vi "FPGA_PWM_dc_motor.vi"(7 "DC PWM Frequency (Hz)":sgl=20000.0, 8 "Encoder Debug":bool, 9 "Loop Timer DAQ":u32=1 caption="Loop Time(uSec)", 10 "Velocity Interval (uSec)":u32=1000, 11 "Controller PWM output [-100,100]%":sgl(slide) scale=-100.0..100.0) -> (0 "Acceleration (Counts/Interval)":i32, 1 "Velocity (Counts/Interval)":i32, 3 "Position (Counts)":i64)   [LabVIEW 2019]
uses:
  <vilib>/rvi/Emulation/niFpgaSctlEmulationGetInTimedLoop.vi
  <vilib>/rvi/Emulation/niFpgaProcessEmulError.vi
  <vilib>/rvi/Emulation/niFpgaGetClockAttributes.vi
  <vilib>/rvi/Emulation/niFpgaEmulationReportErrorSimple.vi
  <vilib>/rvi/eio/common/nirviEmuTemplateMethod_errors.vi
  <vilib>/rvi/Emulation/niFpgaCriticalErrorInLSC.vi
  <vilib>/eio/EIONode/EIONode.xnode
panel:
  out "ConnectorA/DIO13":bool
  out "ConnectorA/DIO12":bool
  in  "Debug: ConnectorA/DIO15":bool
  in  "Debug: ConnectorA/DIO14":bool
  in  "Position Reset":bool
  out "B":bool
  out "A":bool
  out "B'":bool
  out "A'":bool
  in  "stop":bool
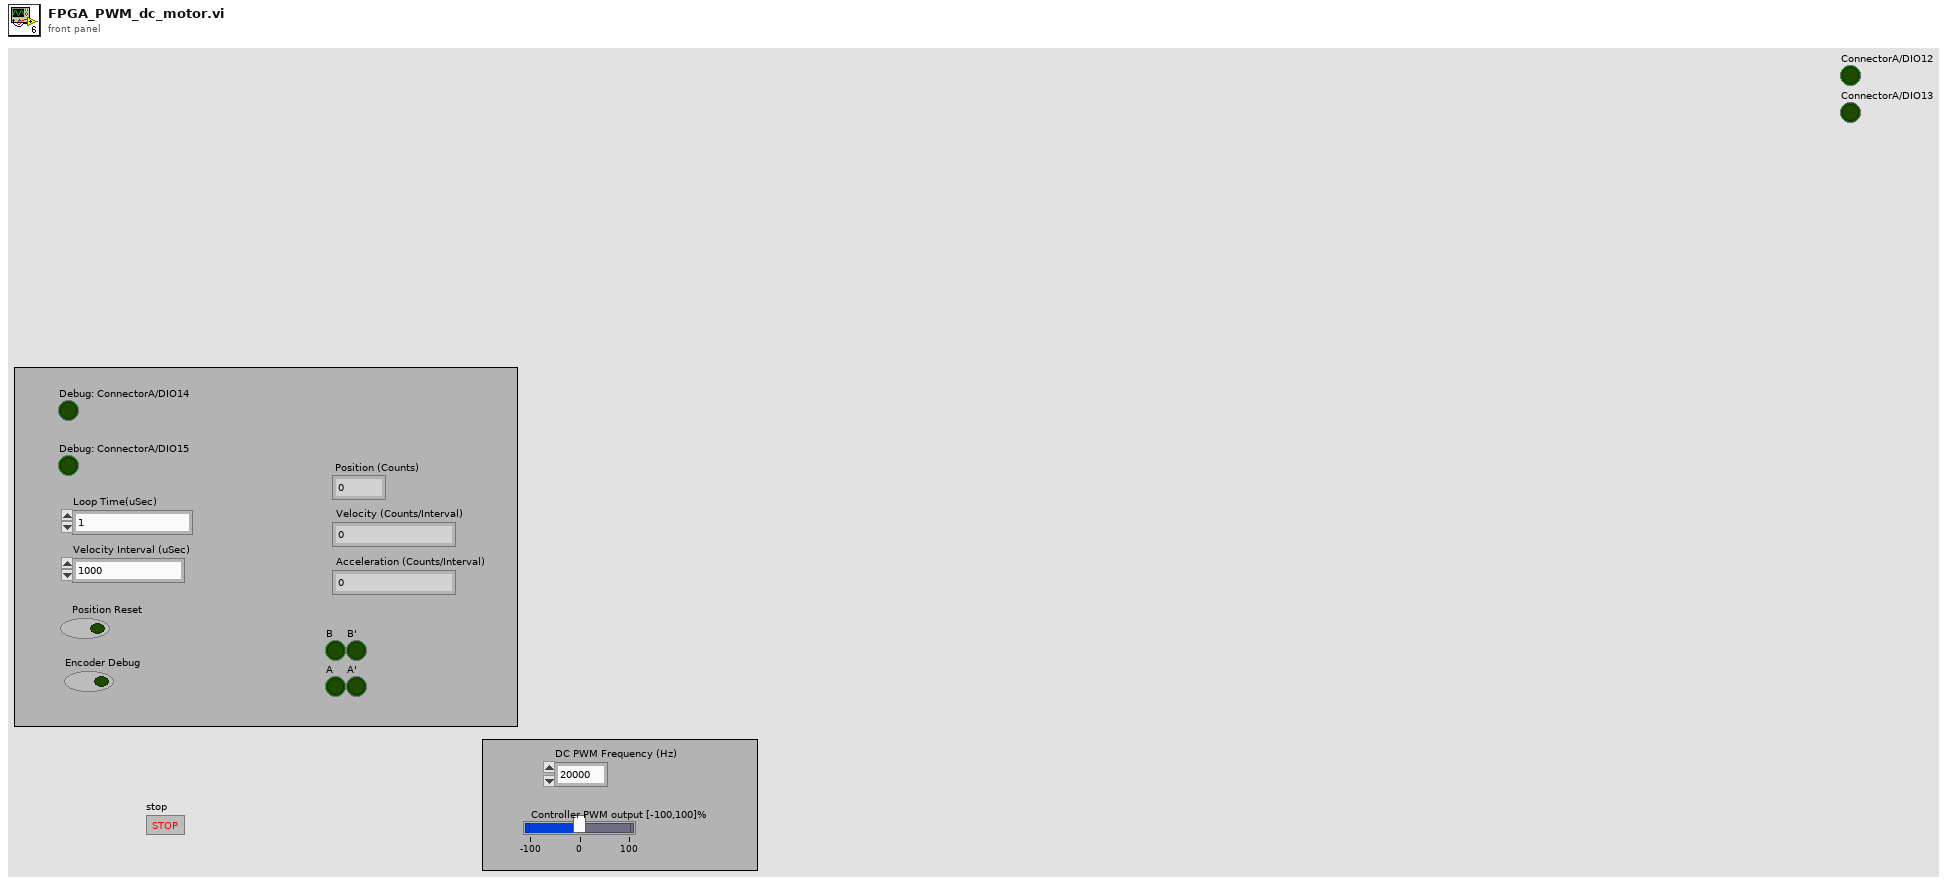
[diagram p1: front panel]
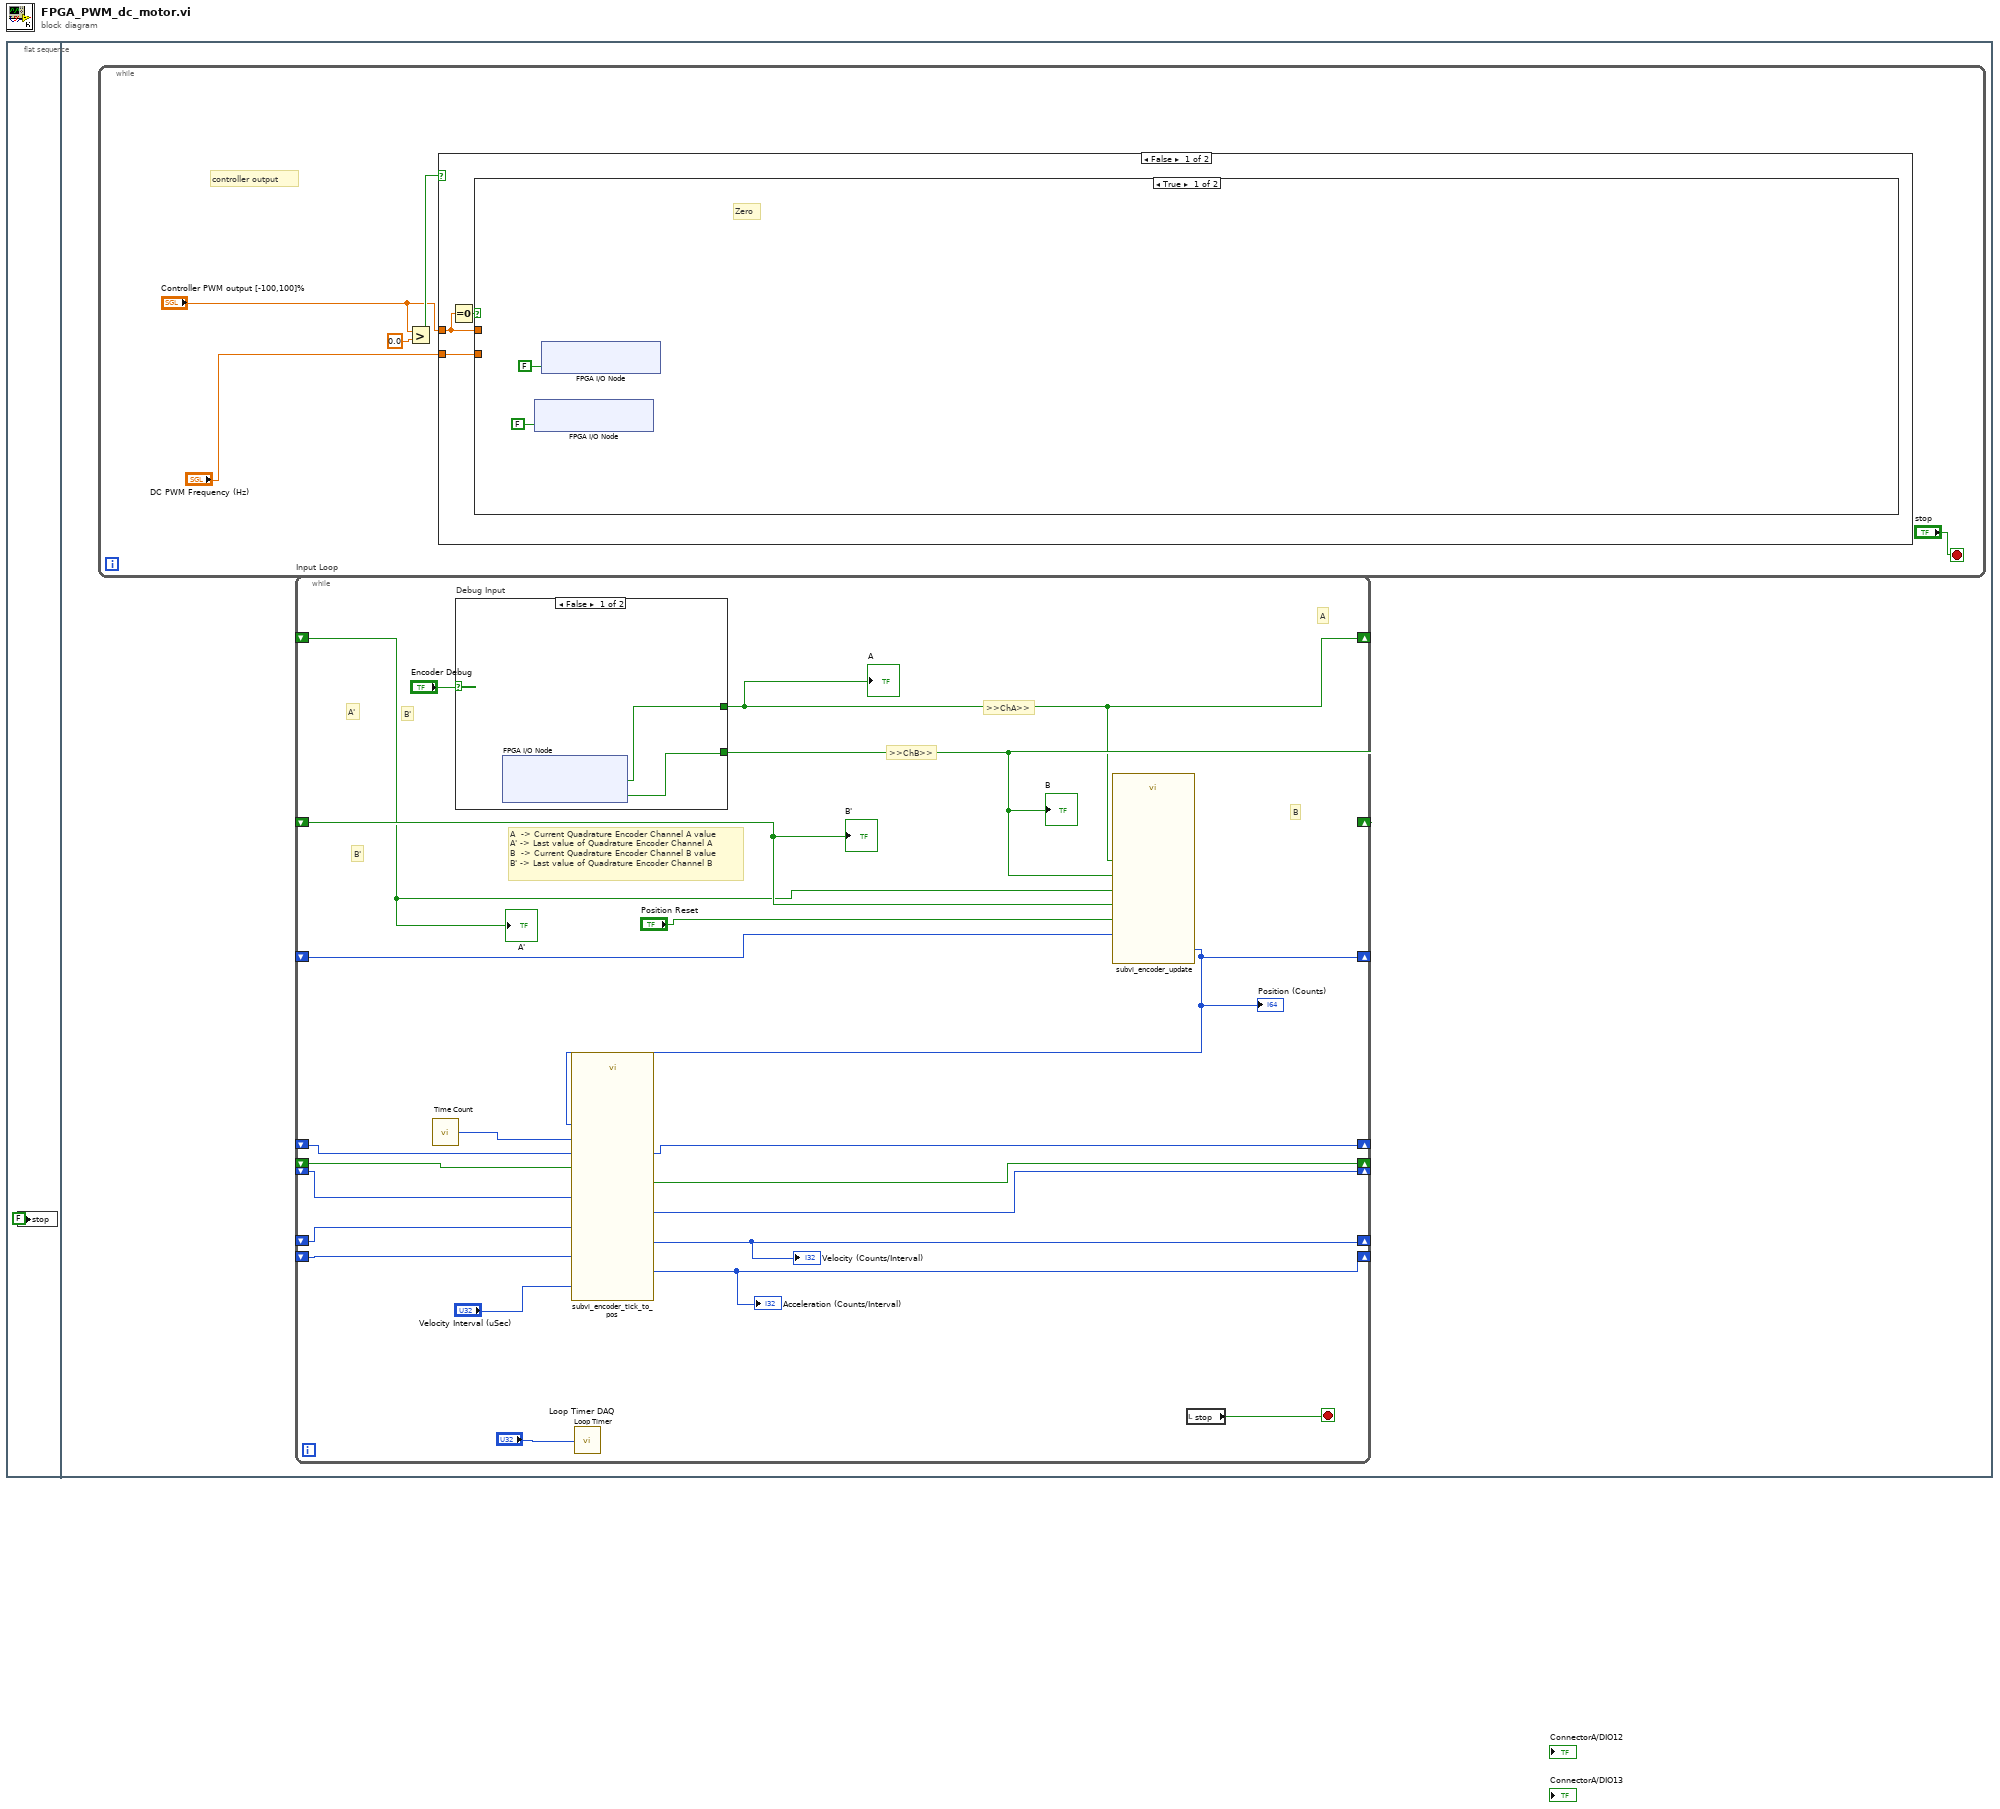
[diagram p0: block diagram]
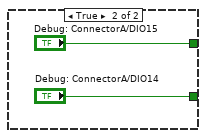
[diagram p2: hidden frame]
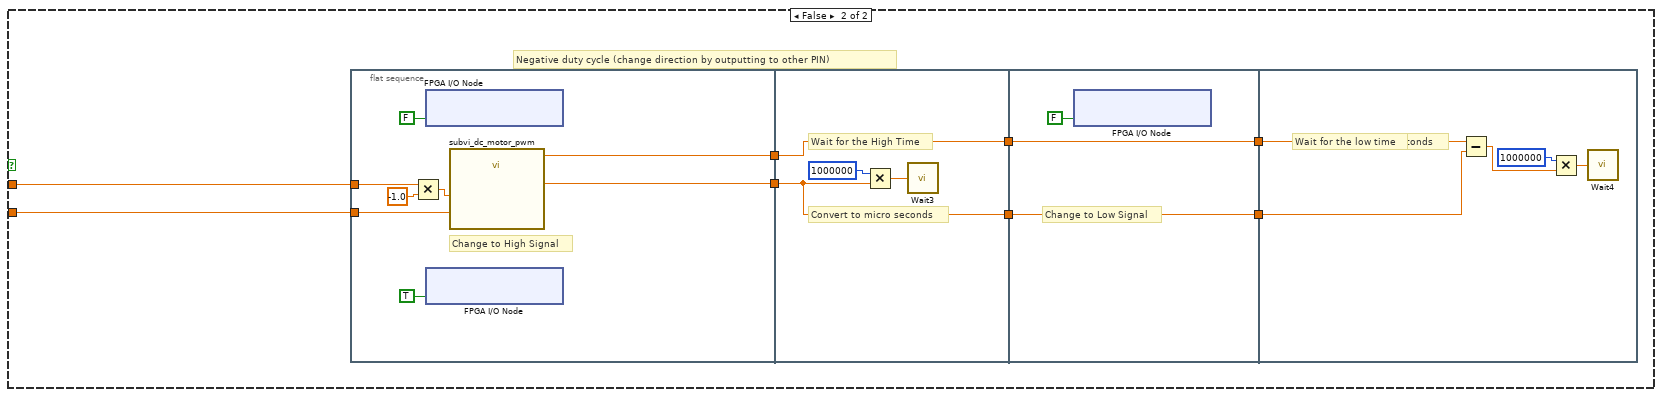
[diagram p3: hidden frame]
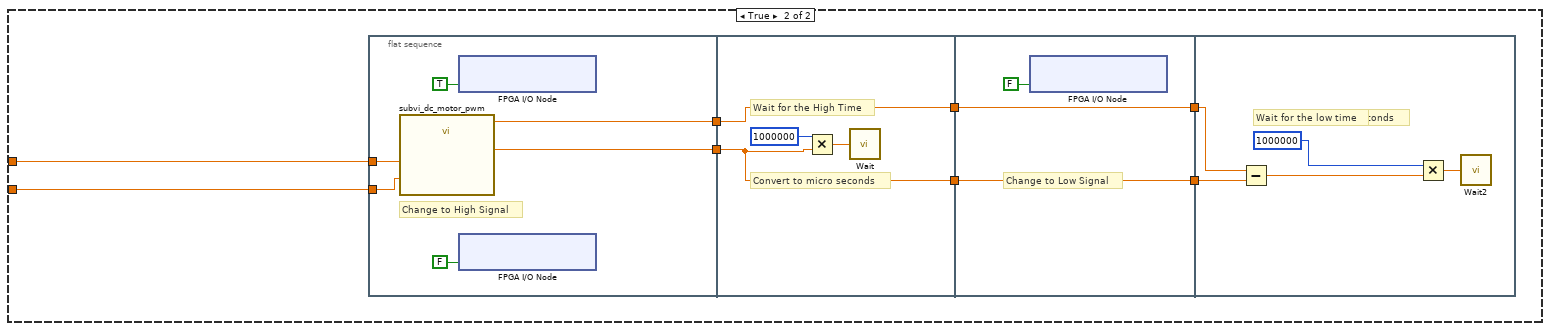
[diagram p4: hidden frame]
diagram:
  n1 = flat-sequence {
    frame #0 {
      n2 = local write "stop"(FALSE ("stop")) -> ()
    }
    frame #1 {
      n3 = while {
        stop <- "stop" stop-if-true
        # "controller output"
        n4 = Greater?(x="Controller PWM output [-100,100]%", y=sgl 0.0) -> (0:w29:bool)
        n5 = case shown="False" w29 {
          tunnel: "DC PWM Frequency (Hz)" -> [w35 w67]
          tunnel: "Controller PWM output [-100,100]%" -> [w34 w66]
          frame False {
            n6 = Equal To 0?(x=w34) -> (x = 0?=w33:bool)
            n7 = case shown="True" w33 {
              tunnel: w34 -> [_ w39]
              tunnel: w35 -> [_ w38]
              frame True {
                # "Zero"
                n8 = xnode "FPGA I/O Node"("ConnectorB/DIO9"=FALSE) -> ()  [unwired: 1 in, 1 out]
                n9 = xnode "FPGA I/O Node"("ConnectorB/DIO8"=FALSE) -> ()  [unwired: 1 in, 1 out]
              }
              frame False {
                # "Negative duty cycle (change direction by outputting to other PIN)"
                n10 = flat-sequence {
                  tunnel: [w52] -> w45
                  tunnel: [w53] -> w44
                  tunnel: w39 -> [w49]
                  tunnel: w38 -> [w47]
                  tunnel: w45 -> [w57]
                  tunnel: [w57] -> w43
                  tunnel: w44 -> [w55]
                  tunnel: [w55] -> w42
                  tunnel: w43 -> [w59]
                  tunnel: w42 -> [w60]
                  tunnel: [w60] -> w41
                  tunnel: [w59] -> w40
                  tunnel: w41 -> [w65]
                  tunnel: w40 -> [w64]
                  frame #0 {
                    # "Change to High Signal"
                    n11 = Multiply(x=w49, y=sgl -1.0) -> (x*y=w48:sgl)
                    n12 = xnode "FPGA I/O Node"("ConnectorB/DIO8"=FALSE) -> ()  [unwired: 1 in, 1 out]
                    n13 = xnode "FPGA I/O Node"("ConnectorB/DIO9"=TRUE) -> ()  [unwired: 1 in, 1 out]
                    n14 = call "subvi_dc_motor_pwm.vi"("Duty Cycle (%)"=w48, "Frequency (Hz)"=w47) -> ("Wait time"=w53:sgl, "Cycle time"=w52:sgl)  [unwired: 8 in]
                  }
                  frame #1 {
                    # "Wait for the High Time"
                    # "Convert to micro seconds"
                    n15 = Multiply(x=u32 1000000, y=w55) -> (x*y=w54:sgl)
                    n16 = call "Wait3"("Count(uSec)"=w54) -> ()  [unwired: 1 out]
                  }
                  frame #2 {
                    # "Change to Low Signal"
                    n17 = xnode "FPGA I/O Node"("ConnectorB/DIO9"=FALSE) -> ()  [unwired: 1 in, 1 out]
                  }
                  frame #3 {
                    # "Convert to micro seconds"
                    # "Wait for the low time"
                    n18 = Subtract(x=w64, y=w65) -> (x-y=w61:sgl)
                    n19 = Multiply(x=u32 1000000, y=w61) -> (x*y=w62:sgl)
                    n20 = call "Wait4"("Count(uSec)"=w62) -> ()  [unwired: 1 out]
                  }
                }
              }
            }
          }
          frame True {
            n21 = flat-sequence {
              tunnel: [w78] -> w73
              tunnel: [w79] -> w72
              tunnel: w67 -> [w76]
              tunnel: w66 -> [w75]
              tunnel: w73 -> [w83]
              tunnel: [w83] -> w71
              tunnel: w72 -> [w81]
              tunnel: [w81] -> w70
              tunnel: w71 -> [w85]
              tunnel: w70 -> [w86]
              tunnel: [w86] -> w69
              tunnel: [w85] -> w68
              tunnel: w69 -> [w91]
              tunnel: w68 -> [w90]
              frame #0 {
                # "Change to High Signal"
                n22 = call "subvi_dc_motor_pwm.vi"("Duty Cycle (%)"=w75, "Frequency (Hz)"=w76) -> ("Wait time"=w79:sgl, "Cycle time"=w78:sgl)  [unwired: 8 in]
                n23 = xnode "FPGA I/O Node"("ConnectorB/DIO8"=TRUE) -> ()  [unwired: 1 in, 1 out]
                n24 = xnode "FPGA I/O Node"("ConnectorB/DIO9"=FALSE) -> ()  [unwired: 1 in, 1 out]
              }
              frame #1 {
                # "Wait for the High Time"
                # "Convert to micro seconds"
                n25 = Multiply(x=u32 1000000, y=w81) -> (x*y=w80:sgl)
                n26 = call "Wait"("Count(uSec)"=w80) -> ()  [unwired: 1 out]
              }
              frame #2 {
                # "Change to Low Signal"
                n27 = xnode "FPGA I/O Node"("ConnectorB/DIO8"=FALSE) -> ()  [unwired: 1 in, 1 out]
              }
              frame #3 {
                # "Convert to micro seconds"
                # "Wait for the low time"
                n28 = Subtract(x=w90, y=w91) -> (x-y=w87:sgl)
                n29 = Multiply(x=u32 1000000, y=w87) -> (x*y=w88:sgl)
                n30 = call "Wait2"("Count(uSec)"=w88) -> ()  [unwired: 1 out]
              }
            }
          }
        }
      }
      n31 = while "Input Loop" {
        shift-right: [w17] -> _
        shift-left: _ -> [w20]
        shift-right: [w16] -> _
        shift-left: _ -> [w19]
        shift-right: [w11] -> _
        shift-left: _ -> [w18]
        shift-right: [w2] -> _
        shift-left: _ -> [w14]
        shift-right: [w3] -> _
        shift-left: _ -> [w13]
        shift-right: [w12] -> _
        shift-left: _ -> [w10]
        shift-right: [w9] -> _
        shift-left: _ -> [w8]
        shift-right: [w7] -> _
        shift-left: _ -> [w6]
        stop <- w4 stop-if-true
        # "B'"
        # ">>ChB>>"
        # ">>ChA>>"
        # "A'"
        # "A  -> Current Quadrature Encoder Channel A value\nA' -> Last value of Quadrature Encoder Channel A\nB  -> Current Quadrature Encoder Channel B value\nB' -> Last value of Quadrature Encoder Channel B"
        # "B'"
        # "B"
        # "A"
        n32 = call "Time Count"() -> ("Tick Count(uSec)"=w5:u32)
        n33 = case "Debug Input" shown="False" "Encoder Debug" {
          tunnel: [w25 "Debug: ConnectorA/DIO15"] -> w16
          tunnel: [w24 "Debug: ConnectorA/DIO14"] -> w17
          frame False {
            n34 = xnode "FPGA I/O Node"() -> ("ConnectorA/DIO12"=w25:bool, "ConnectorA/DIO13"=w24:bool)  [unwired: 2 in, 2 out]
          }
          frame True {
          }
        }
        "B" <- w17
        "A" <- w16
        n35 = call "Loop Timer"("Count(uSec)"="Loop Timer DAQ") -> ()  [unwired: 1 out]
        n36 = call "subvi_encoder_update.vi"("Position Reset"="Position Reset", "Tick'"=w18, "A"=w16, "B'"=w20, "A'"=w19, "B"=w17) -> ("Tick"=w11:i32)  [unwired: 5 in]
        "Position (Counts)" <- w11
        n37 = call "subvi_encoder_tick_to_pos.vi"("Velocity Interval (uSec)"="Velocity Interval (uSec)", "Raw Tick"=w11, "Waited?'"=w8, "Tick Count(uSec)'"=w6, "p'"=w10, "Time Count"=w5, "a'"=w13, "v'"=w14) -> ("Waited?"=w9:bool, "Tick Count(uSec)"=w7:u32, "p"=w12:i32, "a"=w3:i32, "v"=w2:i32)  [unwired: 3 in]
        "Acceleration (Counts/Interval)" <- w3
        "Velocity (Counts/Interval)" <- w2
        n38 = local read "stop"() -> (w4:bool)
        "B'" <- w20
        "A'" <- w19
      }
    }
  }
